vi "biuld_BSON_doc.vi"(6 "innerDoc?(F)":bool, 7 "arrayAsBin(T, x80, T)":T1={"arrayAsBinData"=TRUE, "binDataSubType"=128, "little-endian"=TRUE} {"binDataSubType" format="%02x"}, 8 "error in (no error)":errorcluster, 11 "data":variant) -> (0 "error out":errorcluster, 3 "BSONdoc":u8[](array[numeric]))   [LabVIEW 2015, in "BSON_convertors_Library.lvlib"]
doc: "Created by Artem Shevelev\nLabVIEW Portal profile: http://www.labviewportal.org/memberlist.php?mode=viewprofile&u=2340\ne-mail: artem.sh@gmail.com\nshevelev.pro"
uses:
  BSON_convertors_Library.lvlib
  typedefs/arraySettings_cluster.ctl
  <userlib>/_OpenG.lib/lvdata/lvdata.llb/Type Descriptor Enumeration__ogtk.ctl
  typedefs/dataType.ctl
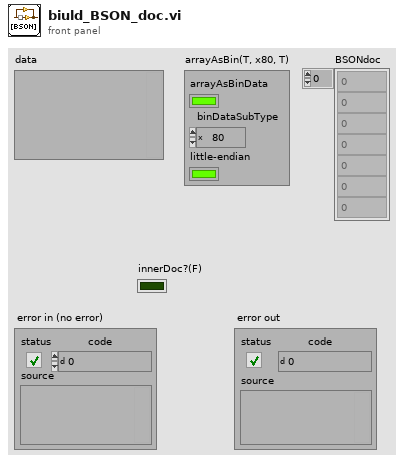
[diagram p1: front panel]
types:
  T1 = typedef "BSON_convertors_Library.lvlib/arraySettings_cluster.ctl" = cluster{"arrayAsBinData":bool, "binDataSubType":u8, "little-endian":bool}
  T2 = typedef "Type Descriptor Enumeration__ogtk.ctl" = enum8{"<Null>", "I8", "I16", "I32", "I64", "U8", "U16", "U32", "U64", "SGL", "DBL", "EXT", "CSG", "CDB", "CXT", "0x0F", "0x10", "0x11", "0x12", "0x13", "0x14", "Enum U8", "Enum U16", "Enum U32", "Enum U64", "SGL PQ", "DBL PQ", "EXT PQ", "CSG PQ", "CDB PQ", "CXT PQ", "0x1F", "0x20", "Boolean", "0x22", "0x23", "0x24", "0x25", "0x26", "0x27", "0x28", "0x29", "0x2A", "0x2B", "0x2C", "0x2D", "0x2E", "0x2F", "String", "0x31", "Path", "Pict", "0x34", "0x35", "0x36", "DAQ", "0x38", "0x39", "0x3A", "0x3B", "0x3C", "0x3D", "0x3E", "0x3F", "Array", "0x41", "0x42", "0x43", "0x44", "0x45", "0x46", "0x47", "0x48", "0x49", "0x4A", "0x4B", "0x4C", "0x4D", "0x4E", "0x4F", "Cluster", "0x51", "0x52", "Variant", "Waveform", "0x55", "0x56", "0x57", "0x58", "0x59", "0x5A", "0x5B", "0x5C", "0x5D", "0x5E", "Fixed Point", "0x60", "0x61", "0x62", "0x63", "0x64", "0x65", "0x66", "0x67", "0x68", "0x69", "0x6A", "0x6B", "0x6C", "0x6D", "0x6E", "0x6F", "Refnum", "0x71", "0x72", "Set Collection", "Map Collection"}
  T3 = typedef "BSON_convertors_Library.lvlib/dataType.ctl" = enum8{"empty(terminator)", "double", "string", "document", "array", "binary", "Deprecated(Undefined)", "ObjectId", "boolean", "UTC datetime", "Null value", "cstring", "Deprecated(DBPointer)", "JavaScript", "Deprecated(Symbol)", "code_w_s", "int32", "uint64", "int64", "ext (decimal128)", "Min key", "Max key"}
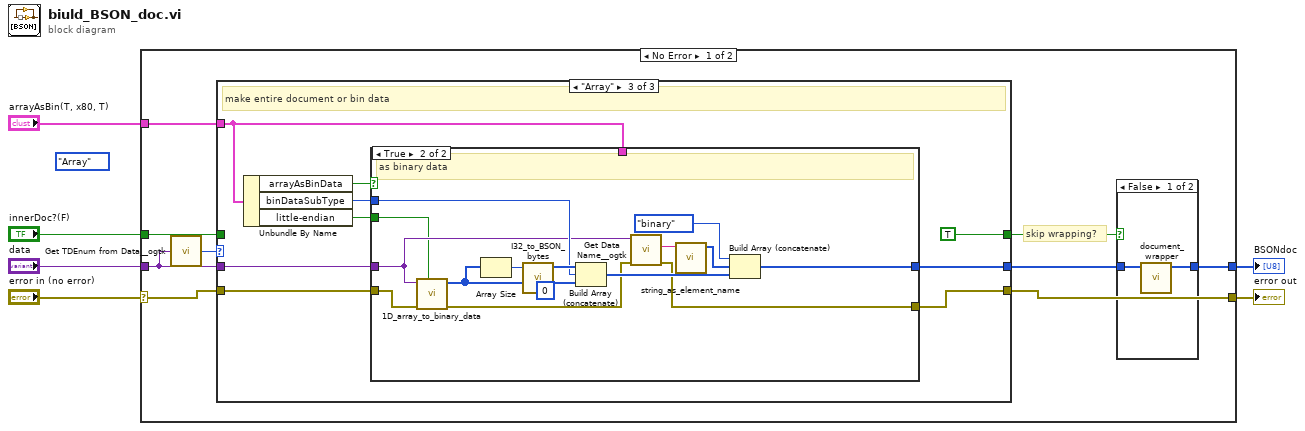
[diagram p0: block diagram]
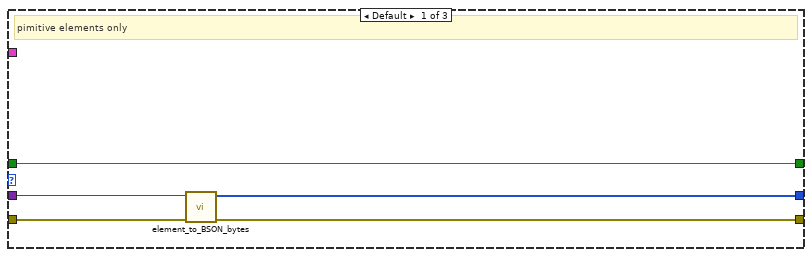
[diagram p3: hidden frame]
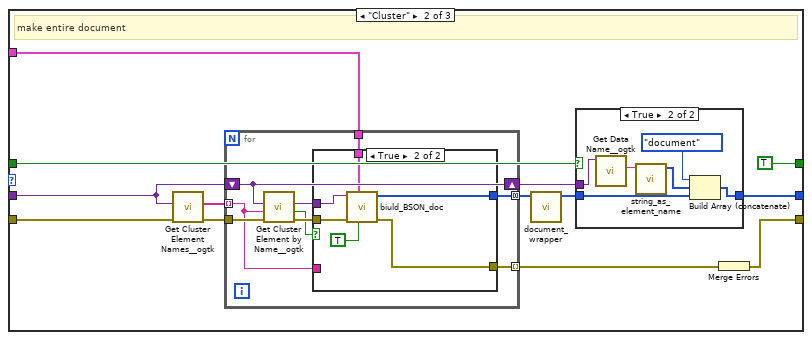
[diagram p4: hidden frame]
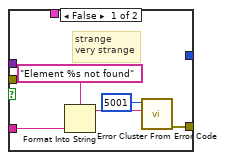
[diagram p6: hidden frame]
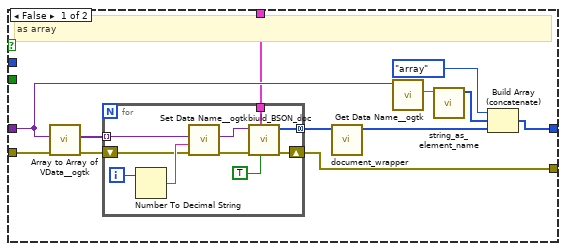
[diagram p7: hidden frame]
diagram:
  (unwired) Type_Descriptor_Enumeration__ogtk."Array" ("Type Descriptor Enumeration")
  n1 = case shown="No Error" "error in (no error)" {
    selector: "error in (no error)" -> [w13 w109]
    tunnel: "data" -> [w14 _]
    tunnel: [w10 w109] -> w6
    tunnel: [w11 _] -> w5
    tunnel: "innerDoc?(F)" -> [w8 _]
    tunnel: "arrayAsBin(T, x80, T)" -> [w7 _]
    frame No Error {
      # "skip wrapping?"
      n2 = call <userlib>:"Get TDEnum from Data__ogtk.vi"("Data"=w14) -> ("Type Descriptor Enumeration"=w15:T2)  [unwired: 4 in]
      n3 = case shown="\"Array\"" w15 {
        tunnel: w14 -> [w23 w33 w68]
        tunnel: [w20 w30 w71] -> w12
        tunnel: w13 -> [w22 w36 w69]
        tunnel: [w21 w31 w72] -> w10
        tunnel: [w19 TRUE ("innerDoc?(F)") TRUE ("innerDoc?(F)")] -> w9
        tunnel: w8 -> [w19 w29 _]
        tunnel: w7 -> [_ w24 w67]
        frame Default {
          # "pimitive elements only"
          n4 = call "element_to_BSON_bytes.vi"("error in (no error)"=w22, "element"=w23) -> ("error out"=w21:errorcluster, "BSONarray"=w20:u8[])  [unwired: 8 in]
        }
        frame "Cluster" {
          # "make entire document"
          n5 = call <userlib>:"Get Cluster Element Names__ogtk.vi"("error in (no error)"=w36, "Cluster"=w33) -> ("error out"=w34:errorcluster, "Element Names"=w35:string[])  [unwired: 8 in]
          n6 = for {
            tunnel: w35 -> [w46] mode=indexing
            tunnel: w34 -> [w52]
            tunnel: [w51] -> w28 mode=concatenating
            tunnel: [w47] -> w32 mode=indexing
            shift-right: [w45] -> w25
            shift-left: w33 -> [w45]
            tunnel: w24 -> [w44]
            n7 = call <userlib>:"Get Cluster Element by Name__ogtk.vi"("error in (no error)"=w52, "Element Name"=w46, "Cluster"=w45) -> ("error out"=w50:errorcluster, "found?"=w48:bool, "VElement"=w49:variant)  [unwired: 6 in]
            n8 = case shown="True" w48 {
              tunnel: [_ w61] -> w51
              tunnel: w50 -> [_ w62]
              tunnel: w49 -> [_ w63]
              tunnel: [w56 w60] -> w47
              tunnel: w46 -> [w54 _]
              tunnel: w44 -> [_ w58]
              frame False {
                # "strange\nvery strange"
                n9 = Format Into String(format string="Element %s not found", w54) -> (resulting string=w53:string)  [unwired: 2 in, 1 out]
                n10 = call <vilib>:"Error Cluster From Error Code.vi"("error message (\"\")"=w53, "error code (0)"=5001) -> ("error out"=w56:errorcluster)  [unwired: 7 in]
              }
              frame True {
                n11 = call "biuld_BSON_doc.vi"("innerDoc?(F)"=TRUE ("skipSimplesWrapper(F)"), "arrayAsBin(T, x80, T)"=w58, "error in (no error)"=w62, "data"=w63) -> ("error out"=w60:errorcluster, "BSONdoc"=w61:u8[])  [unwired: 6 in]
              }
            }
          }
          n12 = call "document_wrapper.vi"("BSONbytes"=w28) -> ("BSONdoc"=w27:u8[])  [unwired: 10 in]
          n13 = case shown="True" w29 {
            tunnel: w27 -> [w37 w43]
            tunnel: [w37 w42] -> w30
            tunnel: w25 -> [_ w38]
            frame False {
            }
            frame True {
              n14 = call <userlib>:"Get Data Name__ogtk.vi"("Data"=w38) -> ("Data Name"=w41:string)  [unwired: 8 in, 2 out]
              n15 = call "string_as_element_name.vi"("result string"=w41) -> ("Array"=w39:u8[])  [unwired: 10 in]
              n16 = Build Array (concatenate)(dataType."document" ("dataType"), w39, w43) -> (w42:u8[])
            }
          }
          n17 = Merge Errors(w32) -> (w31:errorcluster)
        }
        frame "Array" {
          # "make entire document or bin data"
          n18 = Unbundle By Name(w67) -> ("arrayAsBinData"=w66:bool, "binDataSubType"=w65:u8, "little-endian"=w64:bool)
          n19 = case shown="True" w66 {
            tunnel: [w84 w101] -> w72
            tunnel: [w83 w108] -> w71
            tunnel: w69 -> [w79 w99]
            tunnel: w68 -> [w77 w96]
            tunnel: w67 -> [w76 _]
            tunnel: w65 -> [_ w102]
            tunnel: w64 -> [_ w95]
            frame False {
              # "as array"
              n20 = call <userlib>:"Array to Array of VData__ogtk.vi"("error in (no error)"=w79, "MultiD Array"=w77) -> ("error out"=w78:errorcluster, "1D Array of Variants"=w80:variant[])  [unwired: 8 in]
              n21 = for {
                tunnel: [w94] -> w82 mode=concatenating
                tunnel: w80 -> [w91] mode=indexing
                shift-right: [w93] -> w84
                shift-left: w78 -> [w88]
                tunnel: w76 -> [w85]
                i -> [w90]
                n22 = Number To Decimal String(number=w90) -> (decimal integer string=w89:string)  [unwired: 1 in]
                n23 = call <userlib>:"Set Data Name__ogtk.vi"("error in (no error)"=w88, "Data Name"=w89, "Data"=w91) -> ("error out"=w86:errorcluster, "Renamed Data"=w87:variant)  [unwired: 7 in]
                n24 = call "biuld_BSON_doc.vi"("innerDoc?(F)"=TRUE ("skipSimplesWrapper(F)"), "arrayAsBin(T, x80, T)"=w85, "error in (no error)"=w86, "data"=w87) -> ("error out"=w93:errorcluster, "BSONdoc"=w94:u8[])  [unwired: 6 in]
              }
              n25 = call "document_wrapper.vi"("BSONbytes"=w82) -> ("BSONdoc"=w81:u8[])  [unwired: 10 in]
              n26 = call <userlib>:"Get Data Name__ogtk.vi"("Data"=w77) -> ("Data Name"=w75:string)  [unwired: 8 in, 2 out]
              n27 = call "string_as_element_name.vi"("result string"=w75) -> ("Array"=w73:u8[])  [unwired: 10 in]
              n28 = Build Array (concatenate)(dataType."array" ("dataType"), w73, w81) -> (w83:u8[])
            }
            frame True {
              (unwired) u8 0 ("y")
              # "as binary data"
              n29 = call "1D_array_to_binary_data.vi"("little-endian?"=w95, "error in (no error)"=w99, "inputArray"=w96) -> ("error out"=w98:errorcluster, "BSONbytes"=w97:u8[])  [unwired: 7 in]
              n30 = Array Size(array=w97) -> (size(s)=w100:i32)
              n31 = call "I32_to_BSON_bytes.vi"("value"=w100) -> ("BSONbytes"=w107:u8[])  [unwired: 10 in]
              n32 = Build Array (concatenate)(w107, w102, w97) -> (w106:u8[])
              n33 = call <userlib>:"Get Data Name__ogtk.vi"("error in (no error)"=w98, "Data"=w96) -> ("error out"=w101:errorcluster, "Data Name"=w105:string)  [unwired: 7 in, 1 out]
              n34 = call "string_as_element_name.vi"("result string"=w105) -> ("Array"=w103:u8[])  [unwired: 10 in]
              n35 = Build Array (concatenate)(dataType."binary" ("dataType"), w103, w106) -> (w108:u8[])
            }
          }
        }
      }
      n36 = case shown="False" w9 {
        tunnel: w12 -> [w17 w18]
        tunnel: [w16 w18] -> w11
        frame False {
          n37 = call "document_wrapper.vi"("BSONbytes"=w17) -> ("BSONdoc"=w16:u8[])  [unwired: 10 in]
        }
        frame True {
        }
      }
    }
    frame Error {
    }
  }
  "error out" <- w6
  "BSONdoc" <- w5
